vi "Tree-RefreshGeneralTree.vi"(7 "Raw Data From DB Actor":string[][](array[string])=[["PL-2075-3AH", "Manufacturing                                                                                                                                                                                                                                                  ", "1         ", "Testing this crap", "C:\\Users\\tommyj\\Pictures\\ITS ERP System Pictures\\Admin.jpg                                                                                                                                                                                                     ", "C:\\Users\\tommyj\\Pictures\\ITS ERP System Pictures\\Create Inspection Instruction.png                                                                                                                                                                             ", "C:\\Users\\tommyj\\Pictures\\ITS ERP System Pictures\\Stock Inventory.jpg                                                                                                                                                                                           ", "C:\\Users\\tommyj\\Pictures\\ITS ERP System Pictures\\edit-icon.png                                                                                                                                                                                                 ", "C:\\Users\\tommyj\\Pictures\\ITS ERP System Pictures\\Finished Goods Icon.png                                                                                                                                                                                       ", "C:\\Users\\tommyj\\Pictures\\ITS ERP System Pictures\\Pull From Inventory.jpg                                                                                                                                                                                       ", "C:\\Users\\tommyj\\Pictures\\ITS ERP System Pictures\\manufacturing.png                                                                                                                                                                                             ", "Laster Cutting                                                                                                                                                                                                                                                 "], ["PL-2075-3AH", "", "2", "junk", "", "", "", "", "", "", "", ""], ["PL-2075-3AH", "", "3", "asdfasdfasdf", "", "", "", "", "", "", "", ""], ["PP-4562-320", "", "1", "iiiiiiiiii", "", "", "", "", "", "", "", ""], ["PP-4562-320", "", "2", "oooooooooooo", "", "", "", "", "", "", "", ""], ["PP-4562-320", "", "3", "pppppppppp", "", "", "", "", "", "", "", ""], ["PC-258-4561", "", "1", "kkkkkkkkk", "", "", "", "", "", "", "", ""], ["PC-258-4561", "", "2", "lllllllllllllllh", "", "", "", "", "", "", "", ""], ["PC-258-4561", "", "3", "hhhhhhhhhhhh", "", "", "", "", "", "", "", ""], ["PC-258-4561", "", "4", "mmmmmmmmmmmmm", "", "", "", "", "", "", "", ""]], 8 "error in (no error)":errorcluster, 11 "ERP-CreateInstructions in":refnum<class "ERP-CreateInstructions.lvclass">) -> (0 "error out":errorcluster, 3 "ERP-CreateInstructions out":refnum<class "ERP-CreateInstructions.lvclass">)   [LabVIEW 2013, in "ERP-CreateInstructions.lvclass"]
uses:
  ERP-CreateInstructions.lvclass
  ERP-CreateInstructions.lvclass/ERP-CreateInstructions.ctl
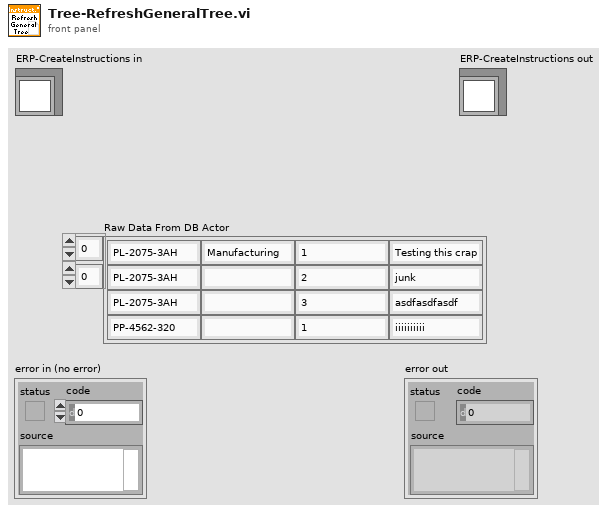
[diagram p1: front panel]
types:
  T1 = cluster{"Left Cell String":string, "Child Text":string[], "Child Tag":string, "Item Indent":i32, "Child Only?":bool, "Glyph Index":i32}[]
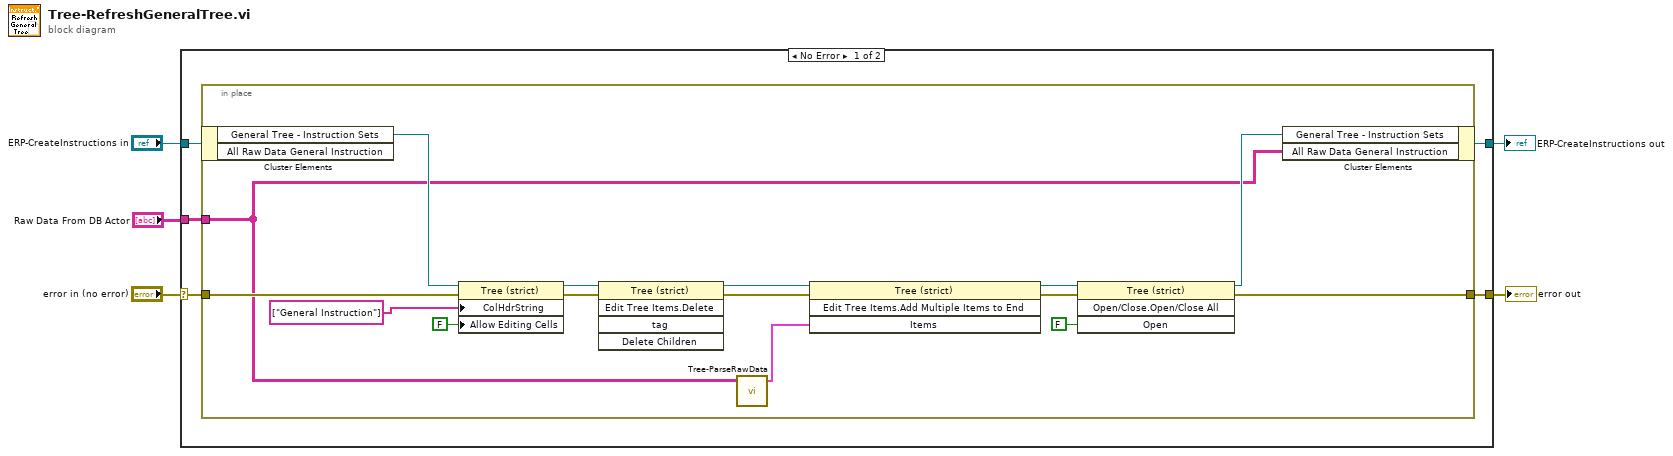
[diagram p0: block diagram]
diagram:
  n1 = case shown="No Error" "error in (no error)" {
    selector: "error in (no error)" -> [w10 w27]
    tunnel: [w9 w27] -> w2
    tunnel: [w7 w26] -> w3
    tunnel: "ERP-CreateInstructions in" -> [w8 w26]
    tunnel: "Raw Data From DB Actor" -> [w6 _]
    frame No Error {
      n2 = in-place {
        in-place-border: w10 -> [w13]
        in-place-border: [w17] -> w9
        in-place-border: w6 -> [w12]
        n3 = in-place-cluster #1(w8) -> ("General Tree - Instruction Sets"=w15:refnum<vi>)  [unwired: 1 out]
        n4 = property on="Property Node" class="Tree (strict)"(reference=w15, error in=w13, "ColHdrString"=string[] ["General Instruction"] ("columns"), "Allow Editing Cells"=FALSE) -> (reference out=w25:refnum<vi>, error out=w24:errorcluster)
        n5 = invoke on="Invoke Node" class="Tree (strict)" method="Edit Tree Items.Delete"(reference=w25, error in=w24) -> (reference out=w20:refnum<vi>, error out=w21:errorcluster)  [unwired: 3 in, 3 out]
        n6 = call "Tree-ParseRawData.vi"("Raw Data"=w12) -> ("Tree Data"=w11:T1)  [unwired: 8 in]
        n7 = invoke on="Invoke Node" class="Tree (strict)" method="Edit Tree Items.Add Multiple Items to End"(reference=w20, error in=w21, "Items"=w11) -> (reference out=w18:refnum<vi>, error out=w19:errorcluster)  [unwired: 1 in, 2 out]
        n8 = invoke on="Invoke Node" class="Tree (strict)" method="Open/Close.Open/Close All"(reference=w18, error in=w19, "Open"=FALSE ("Open?")) -> (reference out=w14:refnum<vi>, error out=w17:errorcluster)  [unwired: 1 in, 2 out]
        n9 = in-place-cluster #1("General Tree - Instruction Sets"=w14, "All Raw Data General Instruction"=w12) -> (w7:refnum<class "ERP-CreateInstructions.lvclass">)
      }
    }
    frame Error {
    }
  }
  "error out" <- w2
  "ERP-CreateInstructions out" <- w3
